vi "CRC-32-IEEE 802.3.vi"(1 "unsigned byte array":u8[](array[numeric]) format="%x") -> (0 "CRC32Value":u32 format="%x")   [LabVIEW 2017]
panel:
  in  "CRC Buffer":u32=4294967295 format="%x"
  # "Init this to 0xFFFFFFFF - can also be\nused to \"carry\" the result from a previous\nCRC to get the CRC of the concatenation."
  # "Default values for testing are 0x49454e44, the IEND chunk code for the PNG standard. Every\nPNG file in the world ends with the CRC of this, 0xAE426082."
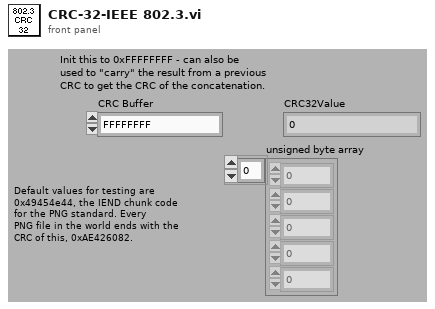
[diagram p1: front panel]
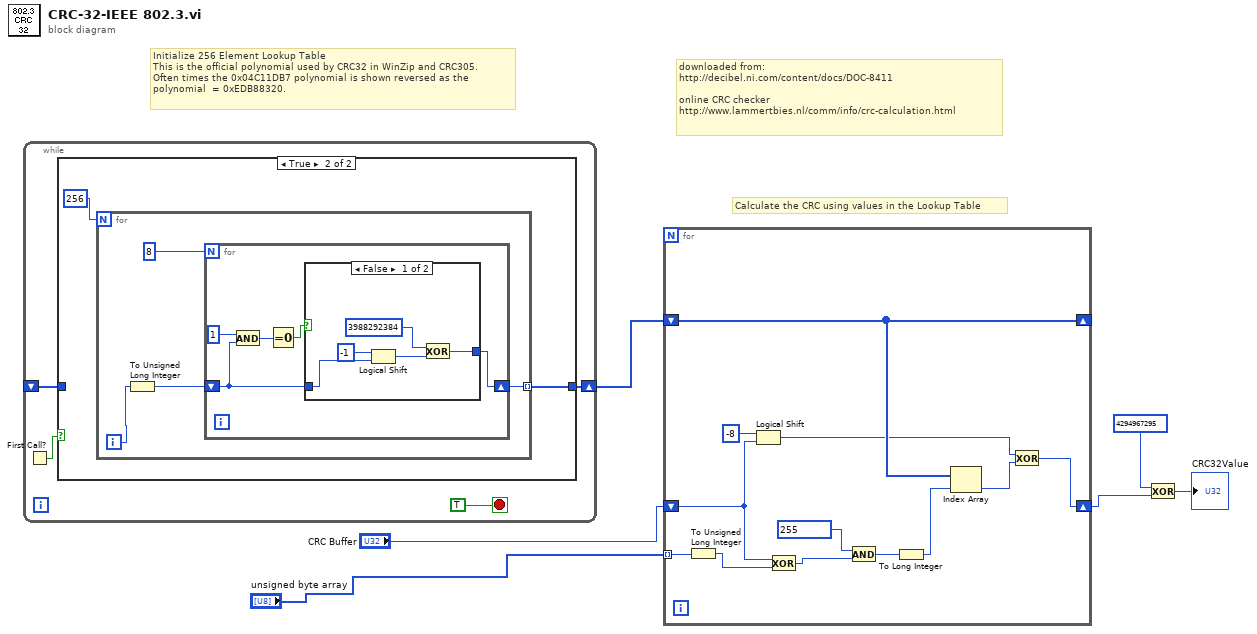
[diagram p0: block diagram]
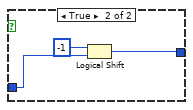
[diagram p3: hidden frame]
diagram:
  # "downloaded from: \nhttp://decibel.ni.com/content/docs/DOC-8411\n\nonline CRC checker\nhttp://www.lammertbies.nl/comm/info/crc-calculation.html"
  # "Calculate the CRC using values in the Lookup Table"
  # "Initialize 256 Element Lookup Table\nThis is the official polynomial used by CRC32 in WinZip and CRC305.\nOften times the 0x04C11DB7 polynomial is shown reversed as the\npolynomial  = 0xEDB88320."
  n1 = while {
    shift-right: [w8] -> w5
    shift-left: _ -> [w7]
    stop <- TRUE stop-if-true
    n2 = First Call?() -> (First Call?: T/F=w9:bool)
    n3 = case shown="True" w9 {
      tunnel: [w11 w12] -> w8
      tunnel: w7 -> [w11 _]
      frame False {
      }
      frame True {
        n4 = for {
          N: 256 -> [_]
          tunnel: [w14] -> w12 mode=indexing
          i -> [w16]
          n5 = To Unsigned Long Integer(number=w16) -> (unsigned 32bit integer=w15:u32)
          n6 = for {
            N: 8 -> [_]
            shift-right: [w18] -> w14
            shift-left: w15 -> [w22]
            n7 = And(x=u32 1, y=w22) -> (x .and. y?=w20:u32)
            n8 = Equal To 0?(x=w20) -> (x = 0?=w19:bool)
            n9 = case shown="False" w19 {
              tunnel: w22 -> [w27 w30]
              tunnel: [w23 w28] -> w18
              frame False {
                n10 = Logical Shift(y=-1, x=w27) -> (x << y=w25:u32)
                n11 = Exclusive Or(1:w25, 2:u32 3988292384 ("x")) -> (0:w23:u32)
              }
              frame True {
                n12 = Logical Shift(y=-1, x=w30) -> (x << y=w28:u32)
              }
            }
          }
        }
      }
    }
  }
  n13 = for {
    tunnel: "unsigned byte array" -> [w37] mode=indexing
    shift-right: [w32] -> w4
    shift-left: "CRC Buffer" -> [w38]
    shift-right: [w42] -> _
    shift-left: w5 -> [w42]
    n14 = To Unsigned Long Integer(number=w37) -> (unsigned 32bit integer=w36:u32)
    n15 = Logical Shift(y=-8, x=w38) -> (x << y=w31:u32)
    n16 = Exclusive Or(1:w36, 2:w38) -> (0:w39:u32)
    n17 = And(x=u32 255, y=w39) -> (x .and. y?=w35:u32)
    n18 = To Long Integer(number=w35) -> (32bit integer=w34:i32)
    n19 = Index Array(array=w42, index=w34) -> (element=w33:u32)
    n20 = Exclusive Or(1:w33, 2:w31) -> (0:w32:u32)
  }
  n21 = Exclusive Or(1:w4, 2:u32 4294967295 ("x")) -> (0:→"CRC32Value":u32)
